vi "Initial Command DAO.vi"(8 "error in (no error)":errorcluster, 9 "Command In":T3, 10 "LBCB Number":T2, 11 "DAO Actions":T1) -> (0 "error out":errorcluster, 1 "Command Out":T3)   [LabVIEW 2013]
uses:
  Data Access Objects/Metadata/Actuator Point.ctl
  Data Access Objects/Metadata/LBCB Number.ctl
  Data Access Objects/Metadata/DAO Actions.ctl
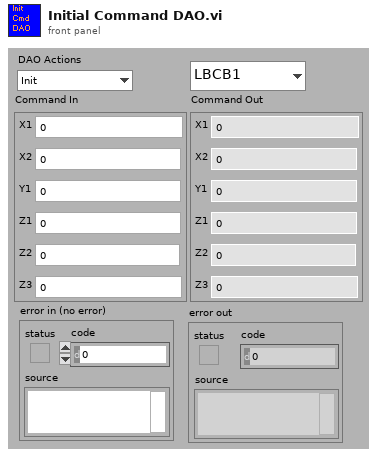
[diagram p1: front panel]
types:
  T1 = typedef "DAO Actions.ctl" = enum16{"Init", "Get", "Set"}
  T2 = typedef "LBCB Number.ctl" = enum16{"LBCB1", "LBCB2"}
  T3 = typedef "Actuator Point.ctl" = cluster{"X1":dbl, "X2":dbl, "Y1":dbl, "Z1":dbl, "Z2":dbl, "Z3":dbl}
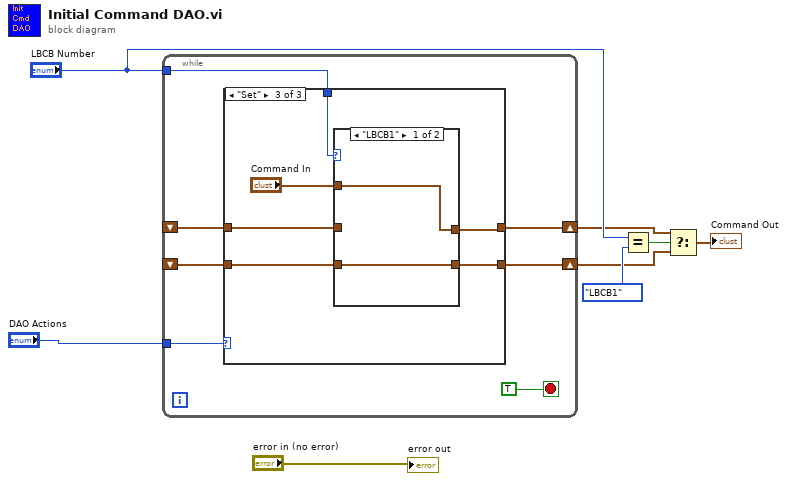
[diagram p0: block diagram]
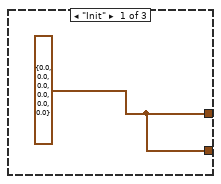
[diagram p2: hidden frame]
diagram:
  n1 = while {
    tunnel: "DAO Actions" -> [w15]
    shift-right: [w14] -> w3
    shift-left: _ -> [w10]
    tunnel: "LBCB Number" -> [w12]
    shift-right: [w11] -> w2
    shift-left: _ -> [w9]
    stop <- TRUE stop-if-true
    n2 = case shown="\"Set\"" w15 {
      tunnel: [w16 w18 w23] -> w14
      tunnel: w12 -> [_ _ w24]
      tunnel: [w16 w17 w21] -> w11
      tunnel: w10 -> [_ w18 w20]
      tunnel: w9 -> [_ w17 w19]
      frame "Init" {
        w16 = T3 {"X1"=0.0, "X2"=0.0, "Y1"=0.0, "Z1"=0.0, "Z2"=0.0, "Z3"=0.0} ("Command In")
      }
      frame "Get" {
      }
      frame "Set" {
        n3 = case shown="\"LBCB1\"" w24 {
          tunnel: [w26 w27] -> w23
          tunnel: "Command In" -> [w26 w28]
          tunnel: [w25 w28] -> w21
          tunnel: w20 -> [_ w27]
          tunnel: w19 -> [w25 _]
          frame "LBCB1" {
          }
          frame "LBCB2" {
          }
        }
      }
    }
  }
  n4 = Equal?(x="LBCB Number", y=LBCB_Number."LBCB1") -> (x = y?=w6:bool)
  n5 = Select(t=w3, s=w6, f=w2) -> (s? t:f=→"Command Out":T3)
  "error out" <- "error in (no error)"
